vi "PMBus Block Process Call.vi"(0 "DevType":i32, 1 "DevIndex":i32, 2 "PMBusIndex":i32, 3 "SlaveAddr":u8, 4 "CommandCode":u8, 5 "pWriteData":string, 6 "WriteByteCount":u8, 7 "error in (no error)":errorcluster, 8 "pReadData":string, 9 "pReadByteCount":string, 10 "PEC":u8) -> (18 "pReadData out":string, 19 "pReadByteCount out":string, 20 "function return":i32, 25 "pWriteData out":string, 27 "error out":errorcluster)   [LabVIEW 2012, in "ControlPMBus.lvlib"]
doc: "int WINAPI PMBus_BlockProcessCall(int DevType,int DevIndex,int PMBusIndex,unsigned char SlaveAddr,unsigned char CommandCode,unsigned char *pWriteData,unsigned char WriteByteCount,unsigned char *pReadData,unsigned char *pReadByteCount,unsigned char PEC);"
uses:
  ControlPMBus.lvlib
  Ginkgo_Driver.dll
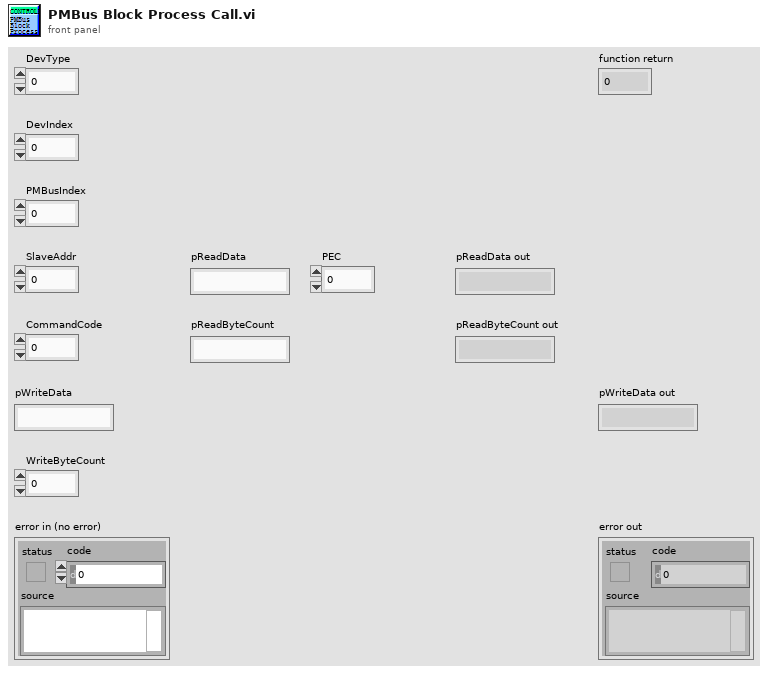
[diagram p1: front panel]
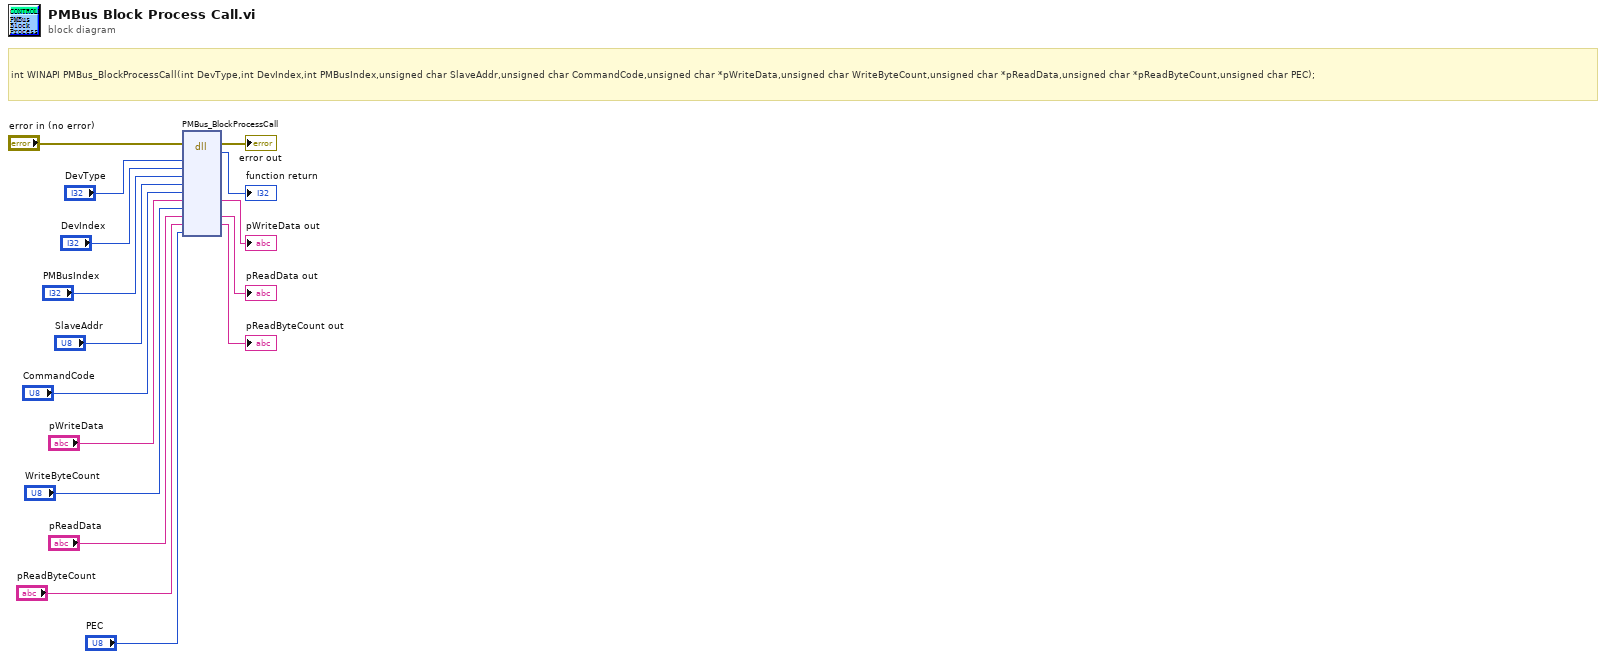
[diagram p0: block diagram]
diagram:
  # "int WINAPI PMBus_BlockProcessCall(int DevType,int DevIndex,int PMBusIndex,unsigned char SlaveAddr,unsigned char CommandCode,unsigned char *pWriteData,unsigned char WriteByteCount,unsigned char *pReadData,unsigned char *pReadByteCount,unsigned char PEC);"
  n1 = dll-call lib="E:/Project/vt_ginkgo/truck/Ginkgo Driver/vs2010/Ginkgo_USB-I2C_API_v2.0.3.0/lib/labview_64bit/ControlPMBus/Ginkgo_Driver.*" fn="PMBus_BlockProcessCall"(error in="error in (no error)", "DevType"="DevType", "DevIndex"="DevIndex", "PMBusIndex"="PMBusIndex", "SlaveAddr"="SlaveAddr", "CommandCode"="CommandCode", "pWriteData"="pWriteData", "WriteByteCount"="WriteByteCount", "pReadData"="pReadData", "pReadByteCount"="pReadByteCount", "PEC"="PEC") -> (error out=→"error out":errorcluster, →"function return":i32, "pWriteData"=→"pWriteData out":string, "pReadData"=→"pReadData out":string, "pReadByteCount"=→"pReadByteCount out":string)  [unwired: 9 in, 1 out]
